vi "SAVE_PATTERN SUB_VI.vi"(9 "PROJECT TITLE":string, 10 "Cluster":cluster{dbl[], dbl[]}) -> ()   [LabVIEW 2017]
uses:
  Control 3.ctl
  Control 2.ctl
  <vilib>/Utility/sysdir.llb/System Directory Type.ctl
  <vilib>/Utility/file.llb/Write Delimited Spreadsheet (DBL).vi
panel:
  in  "?":T1
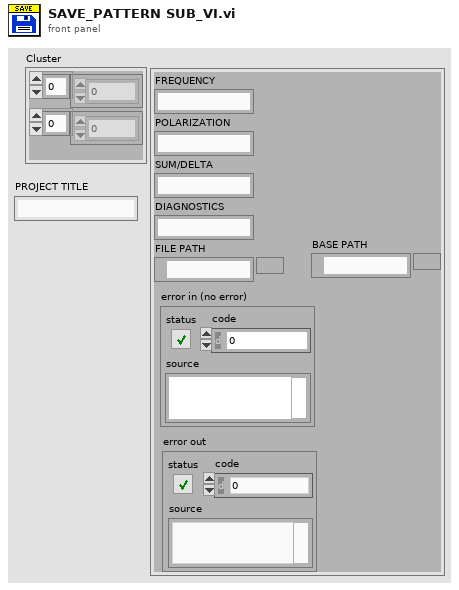
[diagram p1: front panel]
types:
  T1 = typedef "Control 3.ctl" = cluster{"FREQUENCY":string, "POLARIZATION":string, "SUM/DELTA":string, "DIAGNOSTICS":string, "FILE PATH":path, "error in (no error)":errorcluster, "error out":errorcluster, "BASE PATH":path}
  T2 = typedef "Control 2.ctl" = enum16{"STATUS REPORTING", "WRITE CSV FILE", "FILE PATH CHECK", "SAVE DIALOG", "BUILD FILE PATH", "BUILD DIRECTORY PATH", "DIRECTORY PATH CHECK"}
  T3 = typedef "System Directory Type.ctl" = i32
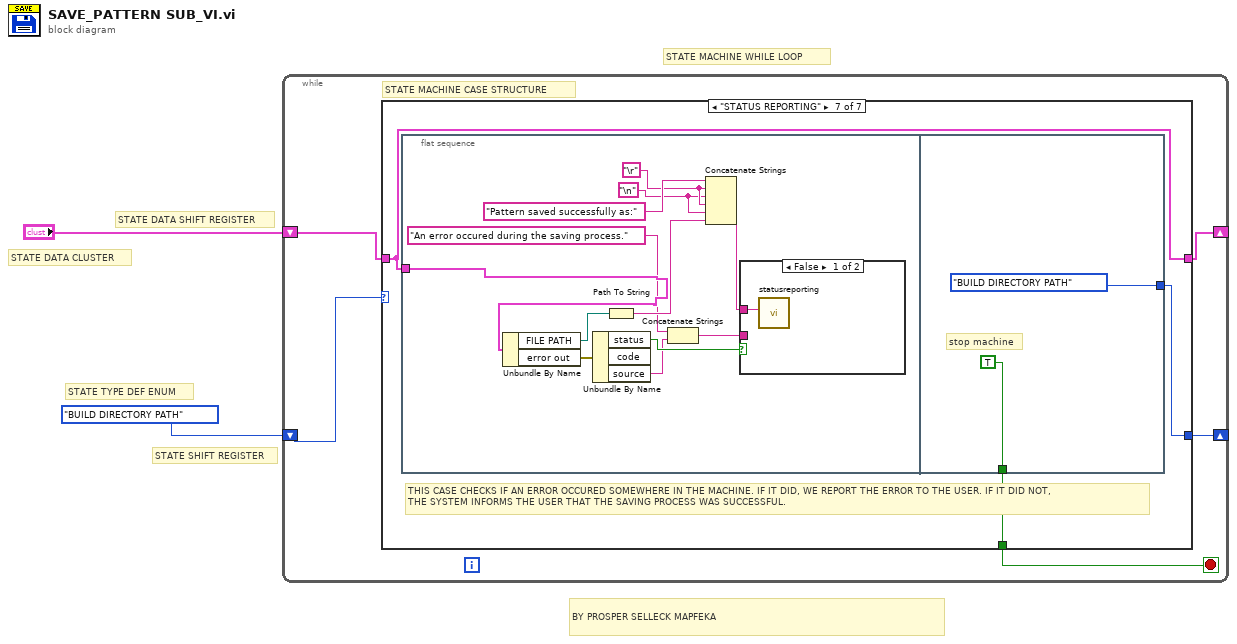
[diagram p0: block diagram]
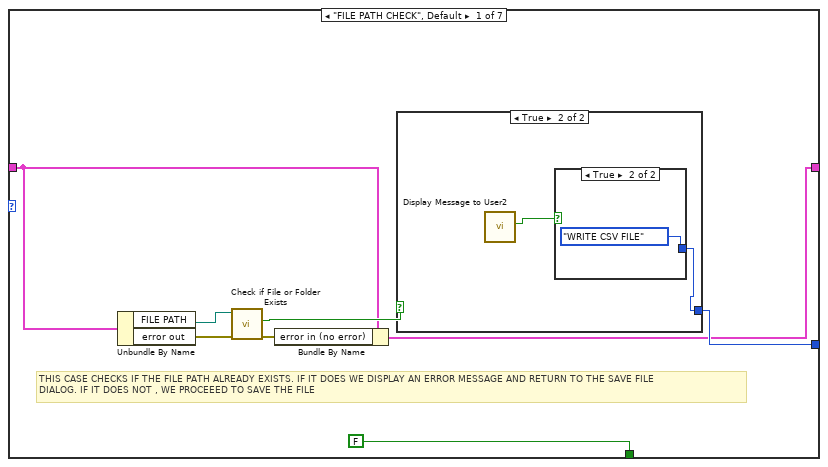
[diagram p2: hidden frame]
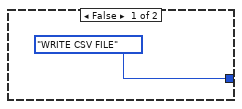
[diagram p3: hidden frame]
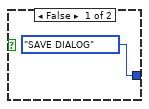
[diagram p4: hidden frame]
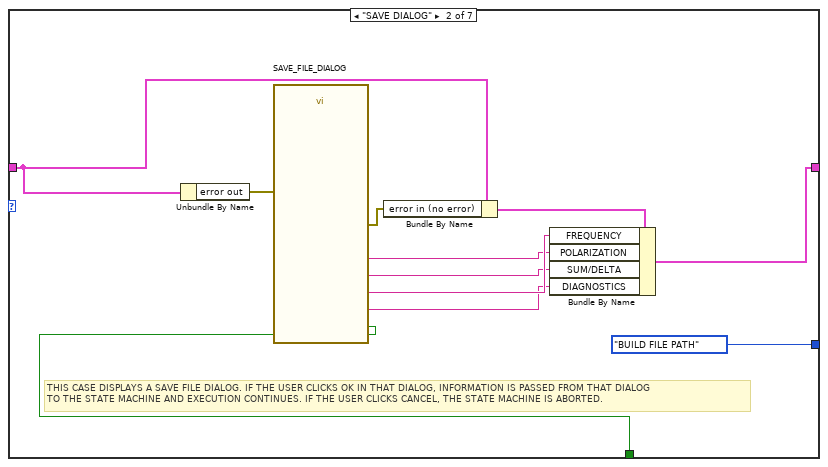
[diagram p5: hidden frame]
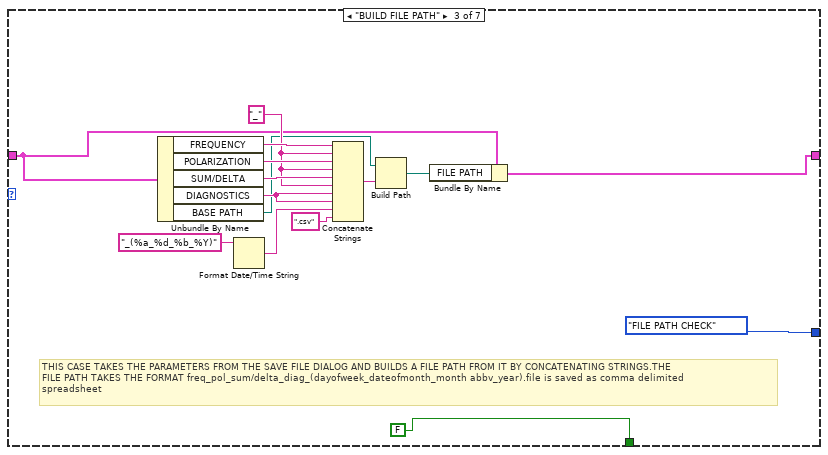
[diagram p6: hidden frame]
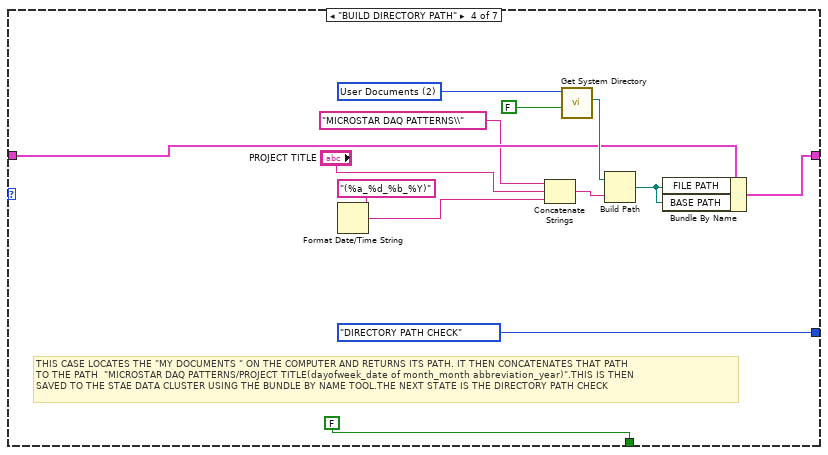
[diagram p7: hidden frame]
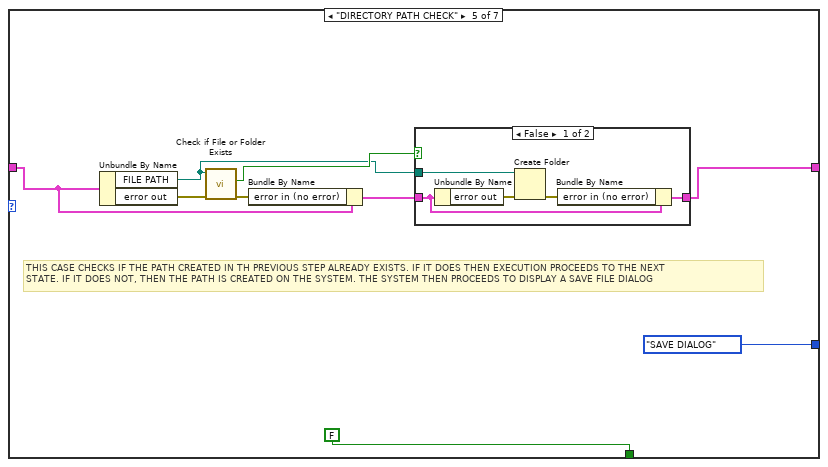
[diagram p8: hidden frame]
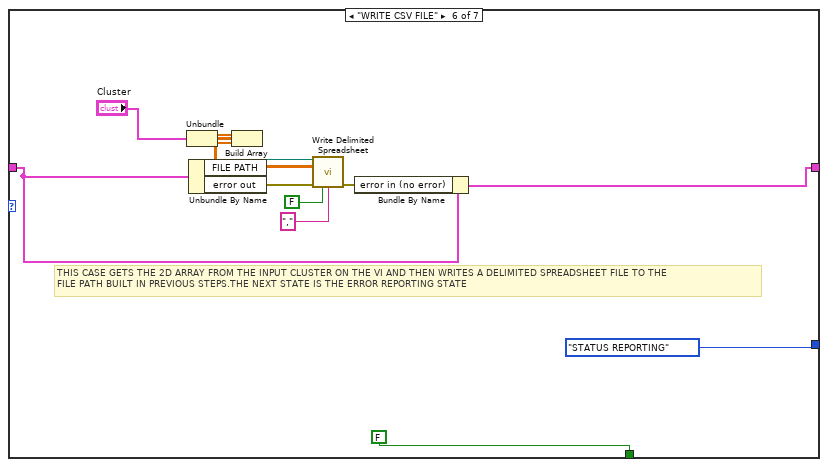
[diagram p10: hidden frame]
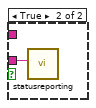
[diagram p11: hidden frame]
diagram:
  # "BY PROSPER SELLECK MAPFEKA"
  # "STATE DATA CLUSTER"
  # "STATE DATA SHIFT REGISTER"
  # "STATE TYPE DEF ENUM"
  # "STATE SHIFT REGISTER"
  # "STATE MACHINE WHILE LOOP"
  n1 = while {
    shift-right: [w3] -> _
    shift-left: Control_2."BUILD DIRECTORY PATH" -> [w7]
    shift-right: [w5] -> _
    shift-left: "?" -> [w6]
    stop <- w4 stop-if-true
    # "STATE MACHINE CASE STRUCTURE"
    n2 = case shown="\"STATUS REPORTING\"" w7 {
      tunnel: [w12 Control_2."BUILD FILE PATH" Control_2."FILE PATH CHECK" Control_2."DIRECTORY PATH CHECK" Control_2."SAVE DIALOG" Control_2."STATUS REPORTING" w88] -> w3
      tunnel: [w9 w30 w34 w50 w65 w76 w90] -> w5
      tunnel: w6 -> [w10 w22 w33 w51 w63 w77 w90]
      tunnel: [FALSE ("Cancel 2") w31 FALSE ("Cancel 2") FALSE ("Cancel 2") FALSE ("Cancel 2") FALSE ("Cancel 2") w89] -> w4
      frame "FILE PATH CHECK", Default {
        # "THIS CASE CHECKS IF THE FILE PATH ALREADY EXISTS. IF IT DOES WE DISPLAY AN ERROR MESSAGE AND RETURN TO THE SAVE FILE \nDIALOG. IF IT DOES NOT , WE PROCEEED TO SAVE THE FILE"
        n3 = Unbundle By Name(w10) -> ("FILE PATH"=w15:path, "error out"=w8:errorcluster)
        n4 = call <vilib>:"Check if File or Folder Exists.vi"("error in (no error)"=w8, "path"=w15) -> ("error out"=w11:errorcluster, "file or folder exists?"=w14:bool)  [unwired: 7 in, 1 out]
        n5 = Bundle By Name(cluster=w10, "error in (no error)"=w11) -> (w9:T1)
        n6 = case shown="True" w14 {
          tunnel: [Control_2."WRITE CSV FILE" w17] -> w12
          frame False {
          }
          frame True {
            n7 = call "Display Message to User2"() -> ("YES"=w18:bool)  [unwired: 10 in, 1 out]
            n8 = case shown="True" w18 {
              tunnel: [Control_2."SAVE DIALOG" Control_2."WRITE CSV FILE"] -> w17
              frame False {
              }
              frame True {
              }
            }
          }
        }
      }
      frame "SAVE DIALOG" {
        # "THIS CASE DISPLAYS A SAVE FILE DIALOG. IF THE USER CLICKS OK IN THAT DIALOG, INFORMATION IS PASSED FROM THAT DIALOG\nTO THE STATE MACHINE AND EXECUTION CONTINUES. IF THE USER CLICKS CANCEL, THE STATE MACHINE IS ABORTED."
        n9 = Unbundle By Name(w22) -> ("error out"=w21:errorcluster)
        n10 = call "SAVE_FILE_DIALOG.vi"("error in (no error)"=w21) -> ("Cancel 2"=w31:bool, "FREQUENCY 2"=w29:string, "SUM/DELTA 2"=w27:string, "POLARIZATION 2"=w28:string, "Diagnostics 3"=w26:string, "error out"=w24:errorcluster)  [unwired: 12 in, 1 out]
        n11 = Bundle By Name(cluster=w22, "error in (no error)"=w24) -> (w23:T1)
        n12 = Bundle By Name(cluster=w23, "FREQUENCY"=w29, "POLARIZATION"=w28, "SUM/DELTA"=w27, "DIAGNOSTICS"=w26) -> (w30:T1)
      }
      frame "BUILD FILE PATH" {
        w42 = "_" ("string")
        # "THIS CASE TAKES THE PARAMETERS FROM THE SAVE FILE DIALOG AND BUILDS A FILE PATH FROM IT BY CONCATENATING STRINGS.THE\nFILE PATH TAKES THE FORMAT freq_pol_sum/delta_diag_(dayofweek_dateofmonth_month abbv_year).file is saved as comma delimited\nspreadsheet"
        n13 = Unbundle By Name(w33) -> ("FREQUENCY"=w45:string, "POLARIZATION"=w44:string, "SUM/DELTA"=w43:string, "DIAGNOSTICS"=w41:string, "BASE PATH"=w36:path)
        n14 = Format Date/Time String(time format string (%c)="_(%a_%d_%b_%Y)") -> (date/time string=w39:string)  [unwired: 2 in]
        n15 = Concatenate Strings(w45, w42, w44, w42, w43, w42, w41, w41, w39, ".csv" ("string")) -> (w37:string)
        n16 = Build Path(base path=w36, name or relative path=w37) -> (appended path=w35:path)
        n17 = Bundle By Name(cluster=w33, "FILE PATH"=w35) -> (w34:T1)
      }
      frame "BUILD DIRECTORY PATH" {
        w54 = T3 2 items=["User Home"=0, "User Desktop"=1, "User Documents"=2, "User Application Data"=3, "User Preferences"=4, "User Temporary"=5, "Public Documents"=6, "Public Application Data"=7, "Public Preferences"=8, "Public Cache"=13, "System Core Libraries"=9, "System Installed Libraries"=10, "Application Files"=11, "Boot Volume Root"=12] ("system directory type")
        # "THIS CASE LOCATES THE \"MY DOCUMENTS \" ON THE COMPUTER AND RETURNS ITS PATH. IT THEN CONCATENATES THAT PATH\nTO THE PATH  \"MICROSTAR DAQ PATTERNS/PROJECT TITLE(dayofweek_date of month_month abbreviation_year)\".THIS IS THEN \nSAVED TO THE STAE DATA CLUSTER USING THE BUNDLE BY NAME TOOL.THE NEXT STATE IS THE DIRECTORY PATH CHECK"
        n18 = Format Date/Time String(time format string (%c)="(%a_%d_%b_%Y)") -> (date/time string=w59:string)  [unwired: 2 in]
        n19 = Concatenate Strings("MICROSTAR DAQ PATTERNS\\" ("string"), "PROJECT TITLE", w59) -> (w57:string)
        n20 = call <vilib>:"Get System Directory.vi"("create directory if not found? (F)"=FALSE, "system directory type"=w54) -> ("system directory"=w56:path)  [unwired: 9 in]
        n21 = Build Path(base path=w56, name or relative path=w57) -> (appended path=w47:path)
        n22 = Bundle By Name(cluster=w51, "FILE PATH"=w47, "BASE PATH"=w47) -> (w50:T1)
      }
      frame "DIRECTORY PATH CHECK" {
        # "THIS CASE CHECKS IF THE PATH CREATED IN TH PREVIOUS STEP ALREADY EXISTS. IF IT DOES THEN EXECUTION PROCEEDS TO THE NEXT \nSTATE. IF IT DOES NOT, THEN THE PATH IS CREATED ON THE SYSTEM. THE SYSTEM THEN PROCEEDS TO DISPLAY A SAVE FILE DIALOG"
        n23 = Unbundle By Name(w63) -> ("FILE PATH"=w66:path, "error out"=w64:errorcluster)
        n24 = call <vilib>:"Check if File or Folder Exists.vi"("error in (no error)"=w64, "path"=w66) -> ("error out"=w62:errorcluster, "file or folder exists?"=w68:bool)  [unwired: 7 in, 1 out]
        n25 = Bundle By Name(cluster=w63, "error in (no error)"=w62) -> (w61:T1)
        n26 = case shown="False" w68 {
          tunnel: w66 -> [w73 _]
          tunnel: w61 -> [w70 w74]
          tunnel: [w71 w74] -> w65
          frame False {
            n27 = Unbundle By Name(w70) -> ("error out"=w69:errorcluster)
            n28 = Create Folder(path (use dialog)=w73, error in=w69) -> (error out=w72:errorcluster)  [unwired: 1 in, 2 out]
            n29 = Bundle By Name(cluster=w70, "error in (no error)"=w72) -> (w71:T1)
          }
          frame True {
          }
        }
      }
      frame "WRITE CSV FILE" {
        # "THIS CASE GETS THE 2D ARRAY FROM THE INPUT CLUSTER ON THE VI AND THEN WRITES A DELIMITED SPREADSHEET FILE TO THE \nFILE PATH BUILT IN PREVIOUS STEPS.THE NEXT STATE IS THE ERROR REPORTING STATE"
        n30 = Unbundle("Cluster") -> (w82:dbl[], w83:dbl[])
        n31 = Unbundle By Name(w77) -> ("FILE PATH"=w81:path, "error out"=w79:errorcluster)
        n32 = Build Array(w82, w83) -> (w84:dbl[][])
        n33 = call-poly <vilib>:"Write Delimited Spreadsheet.vi"("file path (dialog if empty)"=w81, "2D data"=w84, "error in (no error)"=w79, "transpose? (no:F)"=FALSE, "delimiter (\\t)"="," ("delimiter (\\t)")) -> ("error out"=w78:errorcluster)  [unwired: 9 in, 1 out]
        n34 = Bundle By Name(cluster=w77, "error in (no error)"=w78) -> (w76:T1)
      }
      frame "STATUS REPORTING" {
        # "THIS CASE CHECKS IF AN ERROR OCCURED SOMEWHERE IN THE MACHINE. IF IT DID, WE REPORT THE ERROR TO THE USER. IF IT DID NOT,\nTHE SYSTEM INFORMS THE USER THAT THE SAVING PROCESS WAS SUCCESSFUL."
        n35 = flat-sequence {
          tunnel: w90 -> [w98]
          tunnel: [TRUE] -> w89
          tunnel: [Control_2."BUILD DIRECTORY PATH"] -> w88
          frame #0 {
            w91 = "\n"
            w92 = "\r"
            n36 = Unbundle By Name(w98) -> ("FILE PATH"=w101:path, "error out"=w97:errorcluster)
            n37 = Unbundle By Name(w97) -> ("status"=w96:bool, "source"=w94:string)  [unwired: 1 out]
            n38 = Path To String(path=w101) -> (string=w100:string)
            n39 = Concatenate Strings("An error occured during the saving process." ("string"), w94) -> (w93:string)
            n40 = Concatenate Strings("Pattern saved successfully as:" ("string"), w92, w91, w92, w91, w100) -> (w99:string)
            n41 = case shown="False" w96 {
              tunnel: w99 -> [w103 _]
              tunnel: w93 -> [_ w104]
              frame False {
                n42 = call "statusreporting.vi"("Message"=w103) -> ()  [unwired: 9 in, 2 out]
              }
              frame True {
                n43 = call "statusreporting.vi"("Message"=w104) -> ()  [unwired: 9 in, 2 out]
              }
            }
          }
          frame #1 {
            # "stop machine"
          }
        }
      }
    }
  }
